vi "example.vi"() -> ()   [LabVIEW 2019, in "serial.lvclass"]
uses:
  serial.lvclass
panel:
  in  "串口写入":string
  out "发送返回数":u32
  in  "按钮":bool
  in  "停止":bool
  out "返回数":u32
  out "读取反馈":string
  out "Serial I/O(记录)":refnum<visa-resource-name>
  in  "Serial INI":T1={"VISA串口名称"="COM20", "波特率"=9600, "数据位"=8, "奇偶校验"=enum."None", "停止位"=10, "流控制"=0, "超时"=10000, "终止符"=10, "启用终止符？"=FALSE} {"终止符" format="%.0x"; "流控制" items=["无", "XON/XOFF", "RTS/CTS", "XON/XOFF & RTS/CTS", "DTR/DSR", "XON/XOFF & DTR/DSR"]; "停止位" items=["1.0"=10, "1.5"=15, "2.0"=20]; "数据位" min=5 max=8 step=1}
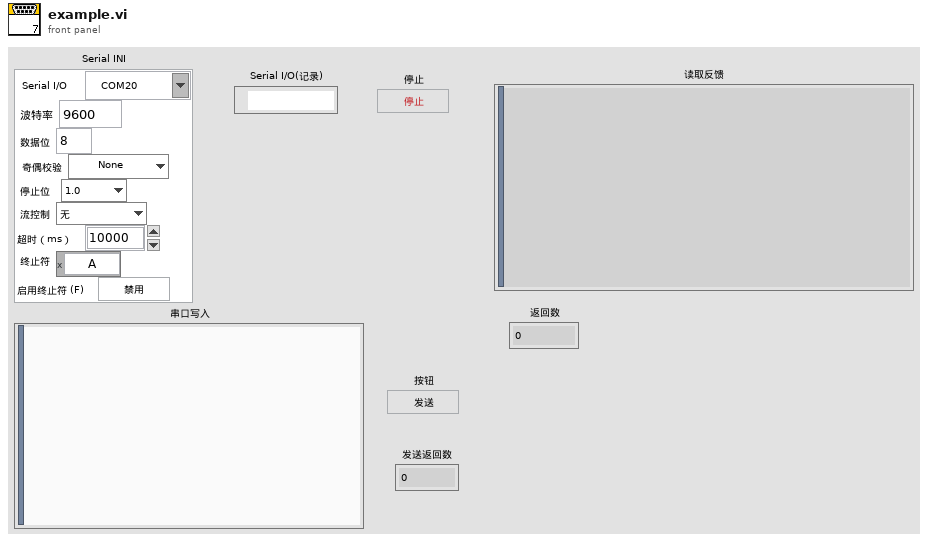
[diagram p1: front panel]
types:
  T1 = cluster{"VISA串口名称":refnum<visa-resource-name>, "波特率":u32, "数据位":u16, "奇偶校验":enum16{"None", "Odd", "Even", "Mark", "Space"}, "停止位":u16, "流控制":u16, "超时":u32, "终止符":u8, "启用终止符？":bool}
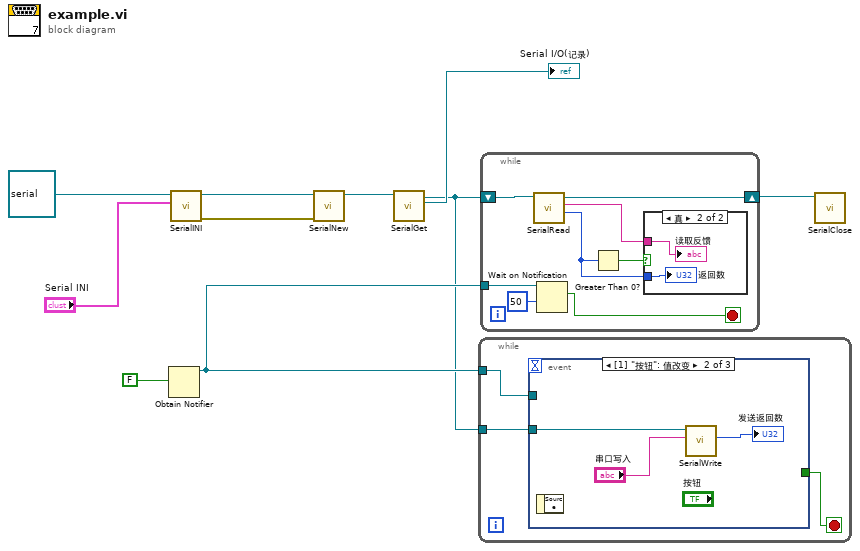
[diagram p0: block diagram]
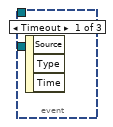
[diagram p3: hidden frame]
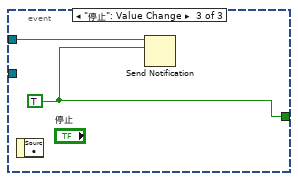
[diagram p4: hidden frame]
diagram:
  n1 = Obtain Notifier(notification data type=FALSE) -> (notifier out=w2:refnum<notifier>)  [unwired: 3 in, 2 out]
  n2 = call-dynamic "SerialINI.vi"("Serial INI"="Serial INI", "serial 输入"=refnum<class "serial.lvclass"> refnum ("serial.lvclass")) -> ("error out"=w7:errorcluster, "serial 输出"=w9:refnum<class "serial.lvclass">)  [unwired: 8 in]
  n3 = call-dynamic "SerialNew.vi"("error in (no error)"=w7, "serial 输入"=w9) -> ("serial 输出"=w6:refnum<class "serial.lvclass">)  [unwired: 7 in, 2 out]
  n4 = call-dynamic "SerialGet.vi"("serial 输入"=w6) -> ("Serial I/O(记录)"=→"Serial I/O(记录)":refnum<visa-resource-name>, "serial 输出"=w1:refnum<class "serial.lvclass">)  [unwired: 8 in, 1 out]
  n5 = while {
    tunnel: w2 -> [w12]
    tunnel: w1 -> [w11]
    stop <- w13 stop-if-true
    n6 = event shown="[1] \"按钮\": 值改变" {
      selector: _ -> [_ _ _]
      dyn-events: _ -> [_ _ _]
      timeout: _ -> [_ _ _]
      tunnel: [_ _ w17] -> w13
      tunnel: w12 -> [_ _ w18]
      tunnel: w11 -> [_ w14 _]
      event Timeout {
        n7 = event-data() -> ()  [unwired: 1 in, 3 out]
      }
      event "按钮": Value Change {
        n8 = event-data() -> ()  [unwired: 1 in, 1 out]
        n9 = call-dynamic "SerialWrite.vi"("串口写入"="串口写入", "serial 输入"=w14) -> ("返回数"=→"发送返回数":u32)  [unwired: 7 in, 2 out]
      }
      event "停止": Value Change {
        w17 = TRUE ("通知")
        n10 = event-data() -> ()  [unwired: 1 in, 1 out]
        n11 = Send Notification(notification=w17, notifier=w18) -> ()  [unwired: 1 in, 2 out]
      }
    }
  }
  n12 = while {
    shift-right: [w25] -> w4
    shift-left: w1 -> [w26]
    tunnel: w2 -> [w21]
    stop <- w19 stop-if-true
    n13 = call-dynamic "SerialRead.vi"("serial 输入"=w26) -> ("返回数"=w22:u32, "读取反馈"=w23:string, "serial 输出"=w25:refnum<class "serial.lvclass">)  [unwired: 7 in, 1 out]
    n14 = Wait on Notification(notifier=w21, timeout in ms (-1)=50 ("超时毫秒(-1)")) -> (notification=w19:bool)  [unwired: 2 in, 3 out]
    n15 = Greater Than 0?(x=w22) -> (x > 0?=w24:bool)
    n16 = case shown="真" w24 {
      tunnel: w23 -> [_ w28]
      tunnel: w22 -> [_ w27]
      frame False {
      }
      frame True {
        "读取反馈" <- w28
        "返回数" <- w27
      }
    }
  }
  n17 = call-dynamic "SerialClose.vi"("serial 输入"=w4) -> ()  [unwired: 9 in, 2 out]
